vi "v2.6.vi"() -> ()   [LabVIEW 2018]
uses:
  <vilib>/DAQmx/read.llb/DAQmx Read (Analog 1D DBL NChan 1Samp).vi
  <extravilib>/ChannelInstances/High Speed Stream-c(a[.](c(dbl,dbl,dbl,dbl)),stamp,a[.](dbl),c(dbl,dbl,dbl,dbl,dbl,dbl,dbl))/_Read For Replicate.vi
  <extravilib>/ChannelInstances/High Speed Stream-c(a[.](c(dbl,dbl,dbl,dbl)),stamp,a[.](dbl),c(dbl,dbl,dbl,dbl,dbl,dbl,dbl))/Instantiate.vi
  <vilib>/Utility/file.llb/Write Delimited Spreadsheet (string).vi
  <extravilib>/ChannelInstances/High Speed Stream-c(a[.](c(dbl,dbl,dbl,dbl)),stamp,a[.](dbl),c(dbl,dbl,dbl,dbl,dbl,dbl,dbl))/)Channel.vi
  <extravilib>/ChannelInstances/High Speed Stream-c(a[.](c(dbl,dbl,dbl,dbl)),stamp,a[.](dbl),c(dbl,dbl,dbl,dbl,dbl,dbl,dbl))/Abort Signal/Init Signal.vi
  <vilib>/DAQmx/create/channels.llb/DAQmx Create Channel (AI-Temperature-Thermocouple).vi
  <vilib>/DAQmx/configure/timing.llb/DAQmx Timing (Sample Clock).vi
  <vilib>/DAQmx/miscellaneous.llb/DAQmx Fill In Error Info.vi
  <extravilib>/ChannelInstances/High Speed Stream-c(a[.](c(dbl,dbl,dbl,dbl)),stamp,a[.](dbl),c(dbl,dbl,dbl,dbl,dbl,dbl,dbl)).lvlib
panel:
  in  "file path (dialog if empty)":path
  out "Enum":T1(ring)
  in  "Start Recording?":bool
  in  "Stop Recording?":bool
  in  "Flowrate Control":dbl
  out "Status":T2(ring)
  in  "OK Button":bool
  in  "DAQ Properties":cluster{"Sample Rate":dbl}={"Sample Rate"=1.0} {"Sample Rate" min=1.0 max=10000.0 step=1.0}
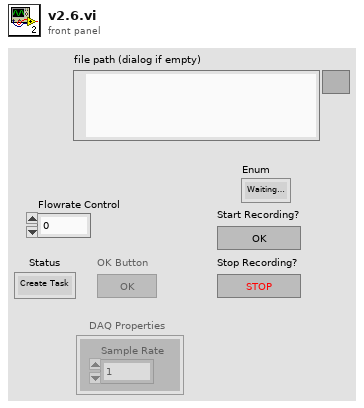
[diagram p1: front panel]
types:
  T1 = enum16{"Waiting to record", "Creating Spreadsheet", "Recording", "Finished Recording"}
  T2 = enum16{"Create Task", "Change Settings", "Check Settings", "Read Data", "End Task"}
  T3 = enum8{"Enabled", "Disabled", "Disabled and Grayed Out"}
  T4 = cluster{"Flowrate Data":cluster{"Line Number":dbl, "Temperature":dbl, "Pressure":dbl, "Flowrate":dbl}[], "Current Time":timestamp, "DAQmx Data":dbl[], "Rig Temperatures":cluster{"BRNR FC":dbl, "BRNR Nozzle":dbl, "Lance Tip":dbl, "Tube 2 Tmp":dbl, "Tube Tmp":dbl, "GA GAS Tmp":dbl, "Chamber External Temp":dbl}}
  T5 = cluster{"BRNR FC":dbl, "BRNR Nozzle":dbl, "Lance Tip":dbl, "Tube 2 Tmp":dbl, "Tube Tmp":dbl, "GA GAS Tmp":dbl, "Chamber External Temp":dbl}
  T6 = cluster{"Line Number":dbl, "Temperature":dbl, "Pressure":dbl, "Flowrate":dbl}[]
  T7 = typedef "High Speed Stream-c(a[.](c(dbl,dbl,dbl,dbl)),stamp,a[.](dbl),c(dbl,dbl,dbl,dbl,dbl,dbl,dbl)).lvlib/)Channel.ctl" = refnum<queue>
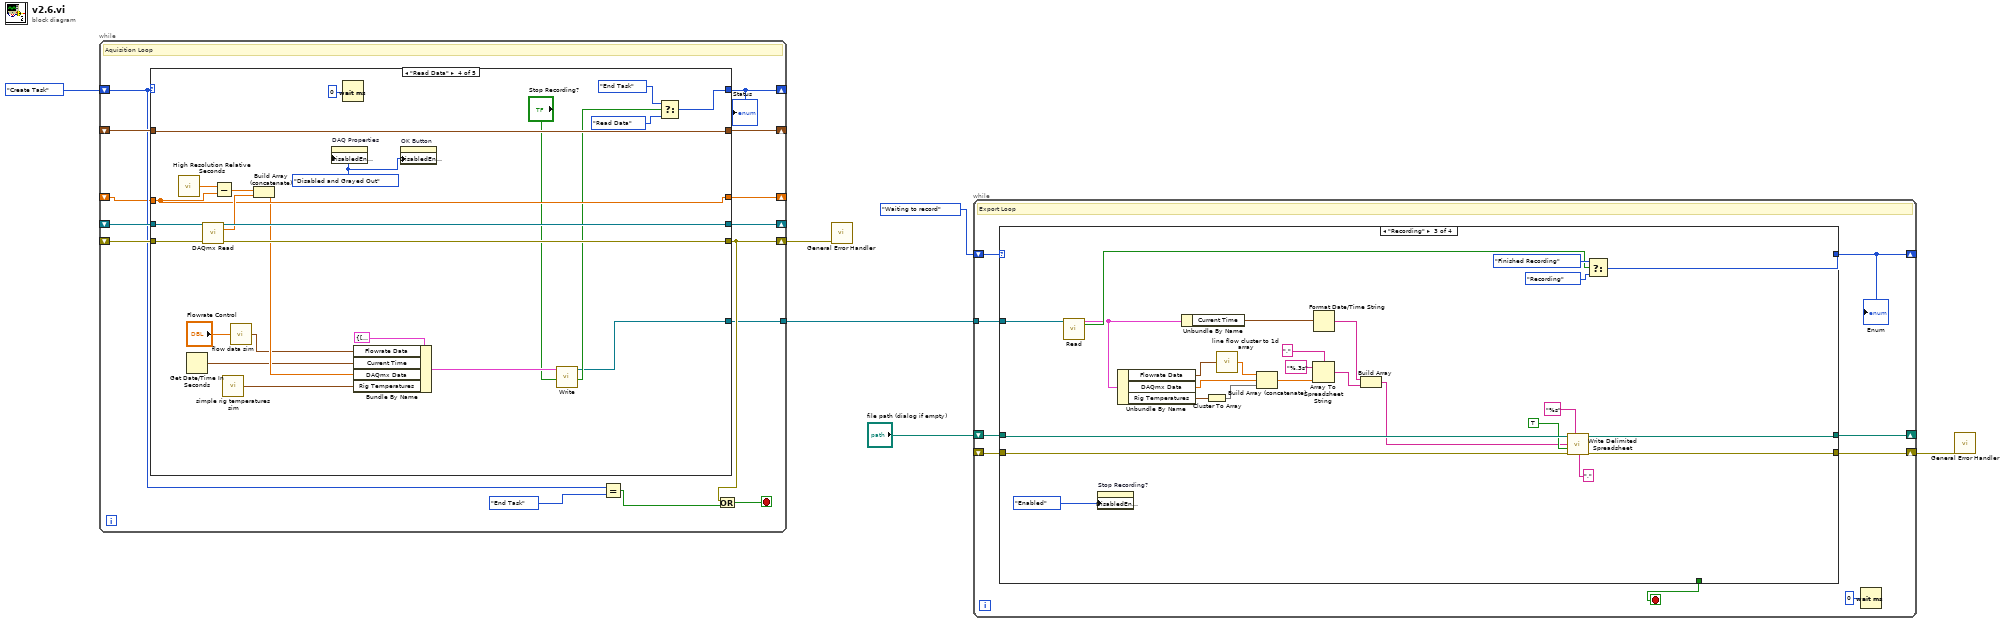
[diagram p0: block diagram]
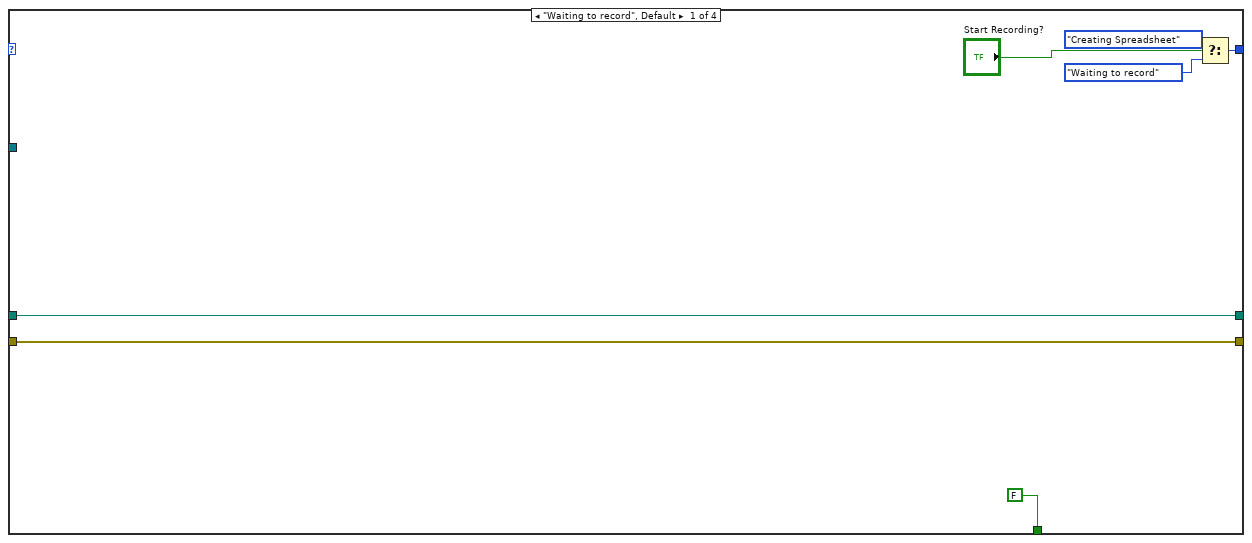
[diagram p2: hidden frame]
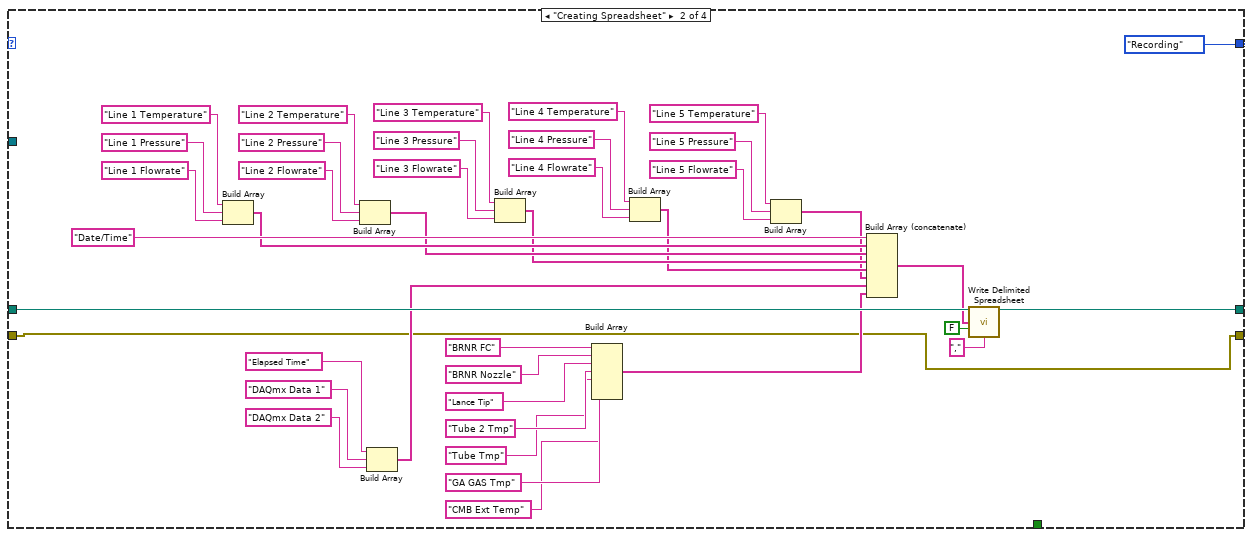
[diagram p3: hidden frame]
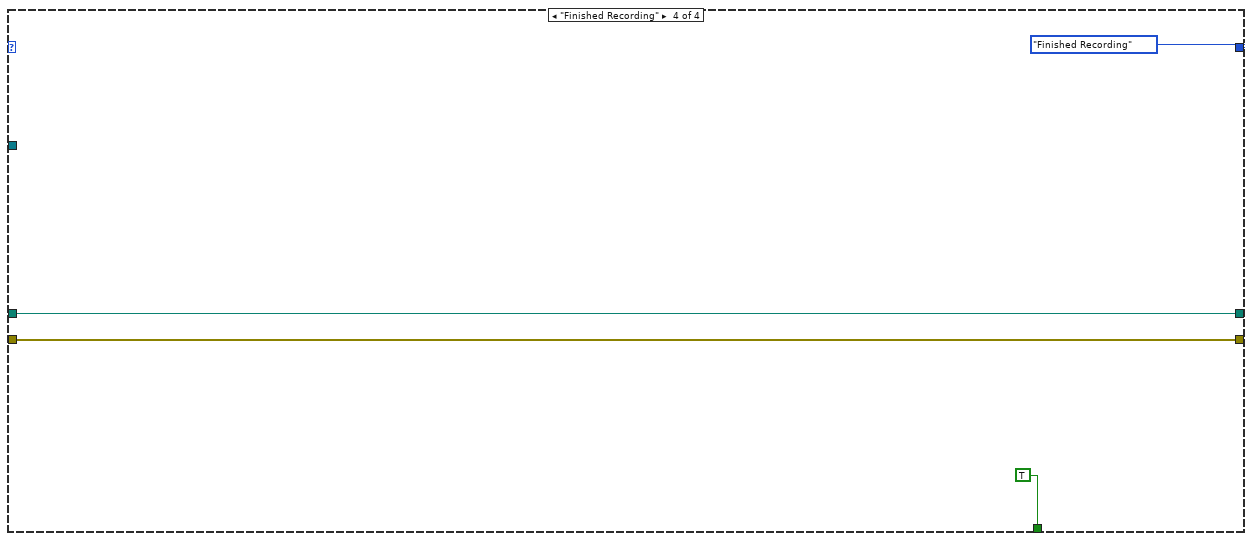
[diagram p4: hidden frame]
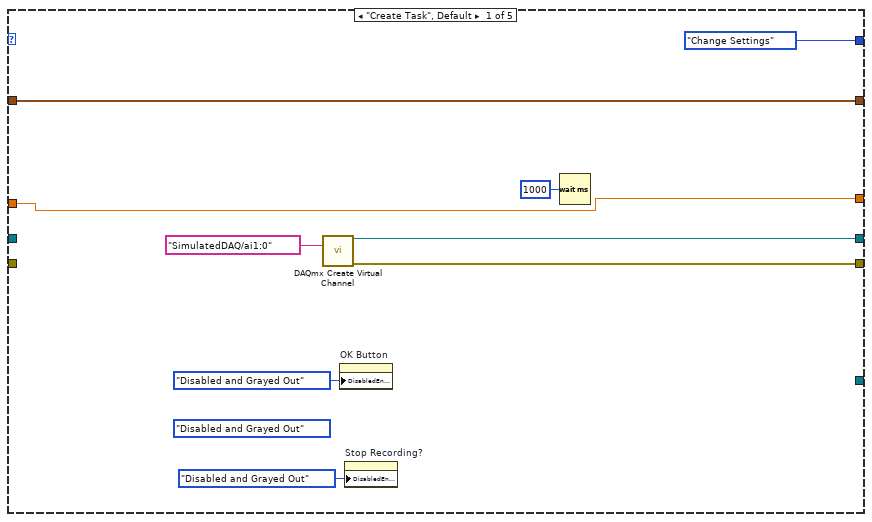
[diagram p5: hidden frame]
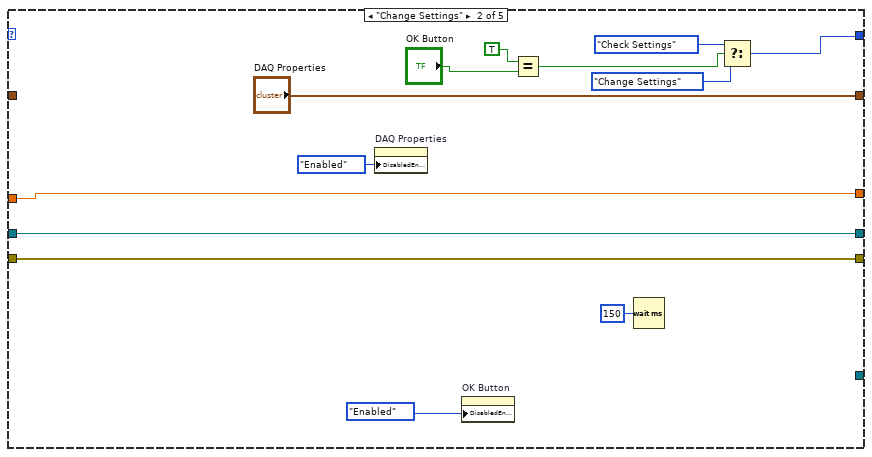
[diagram p6: hidden frame]
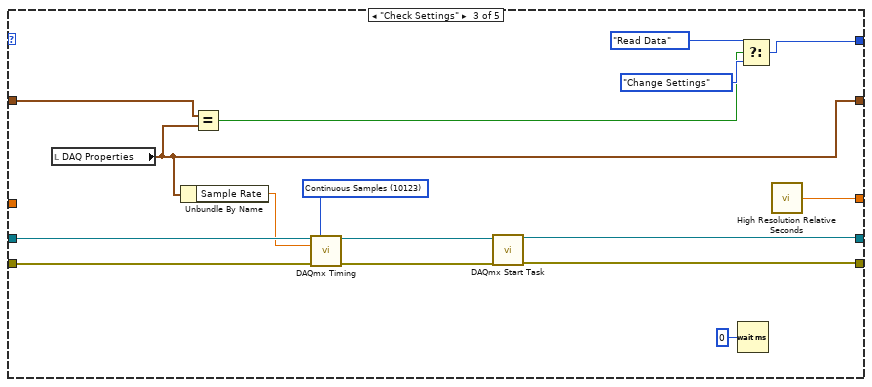
[diagram p7: hidden frame]
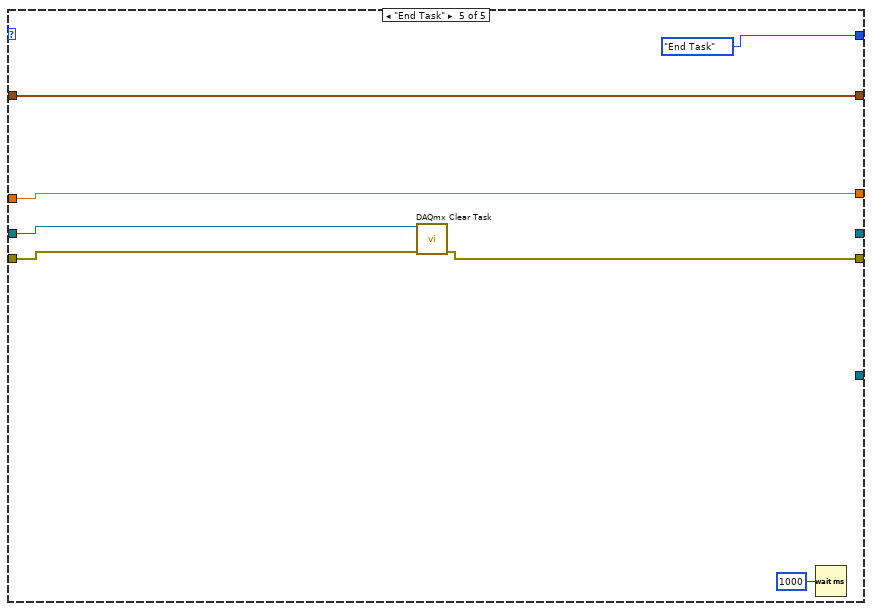
[diagram p8: hidden frame]
diagram:
  n1 = while {
    shift-right: [w15] -> _
    shift-left: T2."Create Task" -> [w11]
    shift-right: [w20] -> _
    shift-left: _ -> [w18]
    shift-right: [w14] -> w1
    shift-left: _ -> [w17]
    shift-right: [w19] -> _
    shift-left: _ -> [w16]
    shift-right: [w10] -> _
    shift-left: _ -> [w9]
    tunnel: [w7] -> w4
    stop <- w8 stop-if-true
    # "Aquisition Loop"
    n2 = case shown="\"Read Data\"" w11 {
      tunnel: [w29 w42 w47 w79 _] -> w20
      tunnel: [w28 w41 w46 w78 w89] -> w14
      tunnel: [T2."Change Settings" w35 w54 w76 T2."End Task"] -> w15
      tunnel: [w25 "DAQ Properties" w50 w80 w88] -> w19
      tunnel: w18 -> [_ w42 w53 w82 w86]
      tunnel: w17 -> [_ w41 w52 w81 w85]
      tunnel: w16 -> [w25 _ w58 w80 w88]
      tunnel: [w23 w32 w43 w70 w84] -> w10
      tunnel: w9 -> [w23 w32 _ w70 w84]
      tunnel: [_ _ _ w59 _] -> w7
      frame "Create Task", Default {
        (unwired) T3."Disabled and Grayed Out" ("Disabled")
        n3 = call-poly <vilib>:"DAQmx Create Virtual Channel.vi"("physical channels"=tag "SimulatedDAQ/ai1:0") -> ("task out"=w29:refnum<k21>, "error out"=w28:errorcluster)  [unwired: 13 in]
        n4 = property on="OK Button" class="Bool"("DisabledEnum"=T3."Disabled and Grayed Out" ("Disabled")) -> ()  [unwired: 2 in, 2 out]
        n5 = property on="Stop Recording?" class="Bool"("DisabledEnum"=T3."Disabled and Grayed Out" ("Disabled")) -> ()  [unwired: 2 in, 2 out]
        n6 = Wait (ms)(milliseconds to wait=u32 1000) -> ()  [unwired: 1 out]
      }
      frame "Change Settings" {
        n7 = property on="DAQ Properties" class="Clust (strict)"("DisabledEnum"=T3."Enabled" ("Disabled")) -> ()  [unwired: 2 in, 2 out]
        n8 = property on="OK Button" class="Bool"("DisabledEnum"=T3."Enabled" ("Disabled")) -> ()  [unwired: 2 in, 2 out]
        n9 = Equal?(x=TRUE, y="OK Button") -> (x = y?=w37:bool)
        n10 = Wait (ms)(milliseconds to wait=u32 150) -> ()  [unwired: 1 out]
        n11 = Select(t=T2."Check Settings", s=w37, f=T2."Change Settings") -> (s? t:f=w35:T2)
      }
      frame "Check Settings" {
        w44 = 10123 items=["Finite Samples"=10178, "Continuous Samples"=10123, "Hardware Timed Single Point"=12522] ("sample mode")
        n12 = local read "DAQ Properties"() -> (w50:cluster{"Sample Rate":dbl})
        n13 = Unbundle By Name(w50) -> ("Sample Rate"=w51:dbl)
        n14 = Equal?(x=w58, y=w50) -> (x = y?=w45:bool)
        n15 = call-poly <vilib>:"DAQmx Timing.vi"("task/channels in"=w53, "sample mode"=w44, "rate"=w51, "error in"=w52) -> ("task out"=w49:refnum<k21>, "error out"=w48:errorcluster)  [unwired: 10 in]
        n16 = call <vilib>:"DAQmx Start Task.vi"("task/channels in"=w49, "error in"=w48) -> ("task out"=w47:refnum<k21>, "error out"=w46:errorcluster)  [unwired: 12 in]
        n17 = Wait (ms)(milliseconds to wait=u32 0) -> ()  [unwired: 1 out]
        n18 = Select(t=T2."Read Data", s=w45, f=T2."Change Settings") -> (s? t:f=w54:T2)
        n19 = call <vilib>:"High Resolution Relative Seconds.vi"() -> ("relative seconds"=w43:dbl)
      }
      frame "Read Data" {
        w68 = T3."Disabled and Grayed Out" ("Disabled")
        n20 = call <vilib>:"High Resolution Relative Seconds.vi"() -> ("relative seconds"=w73:dbl)
        n21 = Get Date/Time In Seconds() -> (seconds since 1Jan1904=w65:timestamp)
        n22 = call-poly <vilib>:"DAQmx Read.vi"("task/channels in"=w82, "error in"=w81) -> ("task out"=w79:refnum<k21>, "data"=w72:dbl[], "error out"=w78:errorcluster)  [unwired: 11 in]
        n23 = Subtract(x=w73, y=w70) -> (x-y=w71:dbl)
        n24 = call "simple rig temperatures sim.vi"() -> ("Rig Temperatures"=w63:T5)
        n25 = call "flow data sim.vi"("Boondoggle Input"="Flowrate Control") -> ("Flowrate Data"=w64:T6)
        n26 = Build Array (concatenate)(w71, w72) -> (w66:dbl[])
        n27 = property on="DAQ Properties" class="Clust (strict)"("DisabledEnum"=w68) -> ()  [unwired: 2 in, 2 out]
        n28 = Wait (ms)(milliseconds to wait=u32 0) -> ()  [unwired: 1 out]
        n29 = Bundle By Name(cluster=T4 {"Flowrate Data"=[{"Line Number"=1.0, "Temperature"=17.480721541683437, "Pressure"=24.0, "Flowrate"=0.0}, {"Line Number"=2.0, "Temperature"=21.850901927104296, "Pressure"=30.0, "Flowrate"=0.0}, {"Line Number"=3.0, "Temperature"=26.221082312525155, "Pressure"=36.0, "Flowrate"=0.0}, {"Line Number"=4.0, "Temperature"=30.591262697946018, "Pressure"=42.00000000000001, "Flowrate"=0.0}, {"Line Number"=5.0, "Temperature"=34.96144308336687, "Pressure"=48.0, "Flowrate"=0.0}], "Current Time"=timestamp(0 s since 1904-01-01), "DAQmx Data"=[], "Rig Temperatures"={"BRNR FC"=0.0, "BRNR Nozzle"=0.0, "Lance Tip"=0.0, "Tube 2 Tmp"=0.0, "Tube Tmp"=0.0, "GA GAS Tmp"=0.0, "Chamber External Temp"=0.0}}, "Flowrate Data"=w64, "Current Time"=w65, "DAQmx Data"=w66, "Rig Temperatures"=w63) -> (w62:T4)
        n30 = property on="OK Button" class="Bool"("DisabledEnum"=w68) -> ()  [unwired: 2 in, 2 out]
        n31 = call <extravilib>:"Write.vi"("last element? (F)"="Stop Recording?", "element"=w62) -> ("done?"=w60:bool, "channel"=w59:T7)  [unwired: 7 in, 1 out]
        n32 = Select(t=T2."End Task", s=w60, f=T2."Read Data") -> (s? t:f=w76:T2)
      }
      frame "End Task" {
        n33 = call <vilib>:"DAQmx Clear Task.vi"("task in"=w86, "error in"=w85) -> ("error out"=w89:errorcluster)  [unwired: 13 in]
        n34 = Wait (ms)(milliseconds to wait=u32 1000) -> ()  [unwired: 1 out]
      }
    }
    "Status" <- w15
    n35 = Equal?(x=w11, y=T2."End Task") -> (x = y?=w12:bool)
    n36 = Or(x=w14, y=w12) -> (x .or. y?=w8:bool)
  }
  n37 = call <vilib>:"General Error Handler.vi"("error in (no error)"=w1) -> ()  [unwired: 10 in, 5 out]
  n38 = while {
    shift-right: [w97] -> _
    shift-left: T1."Waiting to record" -> [w96]
    tunnel: w4 -> [w94]
    shift-right: [w92] -> _
    shift-left: "file path (dialog if empty)" -> [w93]
    shift-right: [w91] -> w2
    shift-left: _ -> [w90]
    stop <- w95 stop-if-true
    # "Export Loop"
    n39 = case shown="\"Recording\"" w96 {
      tunnel: [w102 T1."Recording" w170 T1."Finished Recording"] -> w97
      tunnel: [FALSE _ _ TRUE] -> w95
      tunnel: w94 -> [_ _ w166 _]
      tunnel: w93 -> [w100 w124 w163 w173]
      tunnel: [w100 w123 w164 w173] -> w92
      tunnel: [w99 w106 w152 w172] -> w91
      tunnel: w90 -> [w99 w106 w151 w172]
      frame "Waiting to record", Default {
        n40 = Select(t=T1."Creating Spreadsheet", s="Start Recording?", f=T1."Waiting to record") -> (s? t:f=w102:T1)
      }
      frame "Creating Spreadsheet" {
        n41 = Build Array("Line 1 Temperature", "Line 1 Pressure", "Line 1 Flowrate") -> (w129:string[])
        n42 = Build Array("Line 2 Temperature", "Line 2 Pressure", "Line 2 Flowrate") -> (w128:string[])
        n43 = Build Array("Elapsed Time", "DAQmx Data 1", "DAQmx Data 2") -> (w116:string[])
        n44 = Build Array("Line 3 Temperature", "Line 3 Pressure", "Line 3 Flowrate") -> (w127:string[])
        n45 = Build Array("BRNR FC", "BRNR Nozzle", "Lance Tip", "Tube 2 Tmp", "Tube Tmp", "GA GAS Tmp", "CMB Ext Temp") -> (w108:string[])
        n46 = Build Array("Line 4 Temperature", "Line 4 Pressure", "Line 4 Flowrate") -> (w126:string[])
        n47 = Build Array("Line 5 Temperature", "Line 5 Pressure", "Line 5 Flowrate") -> (w117:string[])
        n48 = Build Array (concatenate)("Date/Time", w129, w128, w127, w126, w117, w116, w108) -> (w122:string[])
        n49 = call-poly <vilib>:"Write Delimited Spreadsheet.vi"("file path (dialog if empty)"=w124, "1D data"=w122, "append to file? (new file:F)"=FALSE, "delimiter (\\t)"="," ("delimiter (\\t)")) -> ("new file path (Not A Path if cancelled)"=w123:path)  [unwired: 10 in, 1 out]
      }
      frame "Recording" {
        n50 = call <extravilib>:"Read.vi"("channel"=w166) -> ("done?"=w165:bool, "element"=w160:T4)  [unwired: 6 in, 3 out]
        n51 = property on="Stop Recording?" class="Bool"("DisabledEnum"=T3."Enabled" ("Disabled")) -> ()  [unwired: 2 in, 2 out]
        n52 = Unbundle By Name(w160) -> ("Flowrate Data"=w161:T6, "DAQmx Data"=w157:dbl[], "Rig Temperatures"=w167:T5)
        n53 = Unbundle By Name(w160) -> ("Current Time"=w159:timestamp)
        n54 = Cluster To Array(cluster=w167) -> (array=w158:dbl[])
        n55 = call "line flow cluster to 1d array.vi"("Flowrate Data"=w161) -> ("Array"=w156:dbl[])
        n56 = Build Array (concatenate)(w156, w157, w158) -> (w155:dbl[])
        n57 = Array To Spreadsheet String(delimiter (Tab)=",", array=w155, 3:"%.3s" ("format string")) -> (spreadsheet string=w146:string)
        n58 = Format Date/Time String(seconds (now)=w159) -> (date/time string=w147:string)  [unwired: 2 in]
        n59 = Build Array(w147, w146) -> (w148:string[])
        n60 = call-poly <vilib>:"Write Delimited Spreadsheet.vi"("file path (dialog if empty)"=w163, "format (%s)"="%s", "1D data"=w148, "append to file? (new file:F)"=TRUE, "error in (no error)"=w151, "delimiter (\\t)"="," ("delimiter (\\t)")) -> ("new file path (Not A Path if cancelled)"=w164:path, "error out"=w152:errorcluster)  [unwired: 8 in]
        n61 = Select(t=T1."Finished Recording", s=w165, f=T1."Recording") -> (s? t:f=w170:T1)
      }
      frame "Finished Recording" {
      }
    }
    "Enum" <- w97
    n62 = Wait (ms)(milliseconds to wait=u32 0) -> ()  [unwired: 1 out]
  }
  n63 = call <vilib>:"General Error Handler.vi"("error in (no error)"=w2) -> ()  [unwired: 10 in, 5 out]
